vi "AnalogIN_Normieren.vi"(7 "Analogwert":sgl, 8 "Obergrenze":sgl, 9 "Untergrenze":sgl, 10 "Max Analogwert":sgl, 11 "Min Analogwert":sgl) -> (0 "Überlauf":bool, 1 "Unterlauf oder Drahtbruch":bool, 2 "Normierter Wert":sgl)   [LabVIEW 2020, in "Verwaltung - cRIO.lvlib"]
uses:
  Verwaltung - cRIO.lvlib
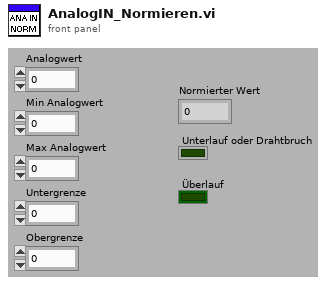
[diagram p1: front panel]
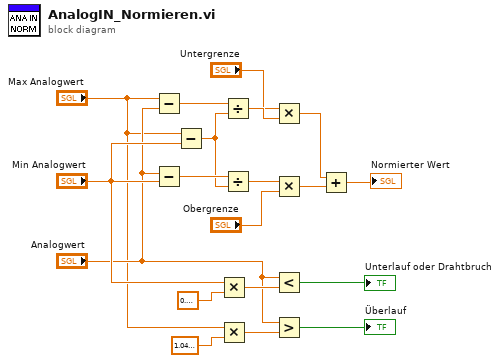
[diagram p0: block diagram]
diagram:
  n1 = Subtract(x="Max Analogwert", y="Analogwert") -> (x-y=w19:sgl)
  n2 = Subtract(x="Analogwert", y="Min Analogwert") -> (x-y=w18:sgl)
  n3 = Subtract(x="Max Analogwert", y="Min Analogwert") -> (x-y=w17:sgl)
  n4 = Multiply(x="Min Analogwert", y=sgl 0.7) -> (x*y=w7:sgl)
  n5 = Multiply(x="Max Analogwert", y=sgl 1.05) -> (x*y=w4:sgl)
  n6 = Divide(x=w19, y=w17) -> (x/y=w16:sgl)
  n7 = Divide(x=w18, y=w17) -> (x/y=w15:sgl)
  n8 = Multiply(x="Untergrenze", y=w16) -> (x*y=w11:sgl)
  n9 = Multiply(x=w15, y="Obergrenze") -> (x*y=w12:sgl)
  n10 = Less?(x="Analogwert", y=w7) -> (x < y?=→"Unterlauf oder Drahtbruch":bool)
  n11 = Greater?(x="Analogwert", y=w4) -> (0:→"Überlauf":bool)
  n12 = Add(x=w11, y=w12) -> (x+y=→"Normierter Wert":sgl)
